vi "Raycaster_CalcWallHeight.vi"(11 "Wall Distance":fxp<+/-,32,16> format="%#_32g") -> (3 "Height Calcs":T1)   [LabVIEW 2020]
uses:
  Controls/Raycaster_ScreenCalcs.ctl
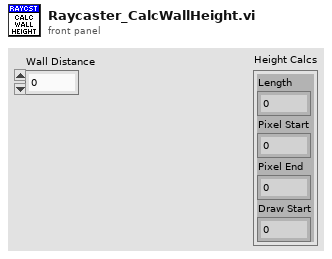
[diagram p1: front panel]
types:
  T1 = typedef "Raycaster_ScreenCalcs.ctl" = cluster{"Length":i16, "Pixel Start":i16, "Pixel End":i16, "Draw Start":i16}
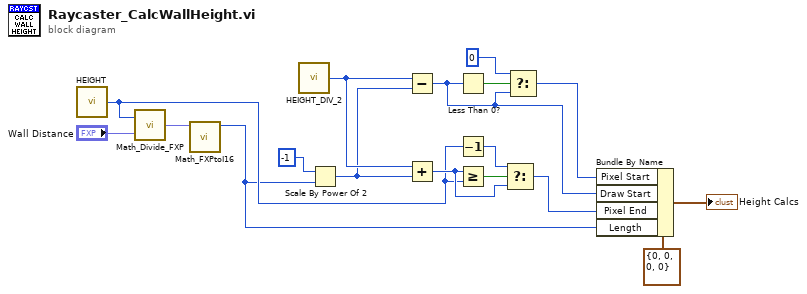
[diagram p0: block diagram]
diagram:
  n1 = call "HEIGHT.vi"() -> ("HEIGHT"=w4:i16)
  n2 = call "Math_Divide_FXP.vi"("y"="Wall Distance", "x"=w4) -> ("x*y"=w5:fxp<+/-,32,16>)
  n3 = call "Math_FXPtoI16.vi"("FXP"=w5) -> ("I16"=w3:i16)  [unwired: 10 in]
  n4 = call "HEIGHT_DIV_2.vi"() -> ("HEIGHT_DIV_2"=w7:i16)
  n5 = Scale By Power Of 2(n=i16 -1, x=w3) -> (x*2^n=w6:i16)
  n6 = Subtract(x=w7, y=w6) -> (x-y=w1:i16)
  n7 = Add(x=w7, y=w6) -> (x+y=w11:i16)
  n8 = Less Than 0?(x=w1) -> (x < 0?=w16:bool)
  n9 = Decrement(x=w4) -> (x-1=w12:i16)
  n10 = Greater Or Equal?(x=w11, y=w4) -> (x >= y?=w13:bool)
  n11 = Select(t=w12, s=w13, f=w11) -> (s? t:f=w8:i16)
  n12 = Select(t=i16 0, s=w16, f=w1) -> (s? t:f=w9:i16)
  n13 = Bundle By Name(cluster=T1 {"Length"=0, "Pixel Start"=0, "Pixel End"=0, "Draw Start"=0} ("Column Calcs"), "Pixel Start"=w9, "Draw Start"=w1, "Pixel End"=w8, "Length"=w3) -> (→"Height Calcs":T1)
